vi "CLSUIP_GrowTermBounds.vi"(1 "Center Point":cluster{"x":i32, "y":i32}, 2 "Multiplication Factor":cluster{"x":i32, "y":i32}, 3 "Terminal Bounds":T1) -> (0 "Grown Bounds":T1)   [LabVIEW 2021, in "MemberVICreation.lvlib" / "VIRetooler.lvclass"]
uses:
  <resource>/Framework/Providers/LVClassLibrary/NewAccessors/VIRetooler/VIRetooler.lvclass
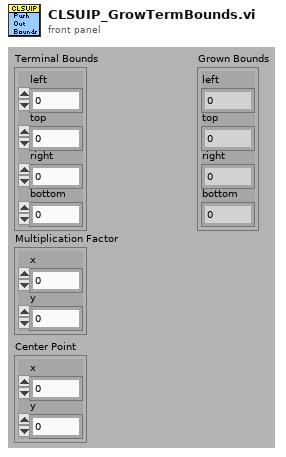
[diagram p1: front panel]
types:
  T1 = cluster{"left":i16, "top":i16, "right":i16, "bottom":i16}
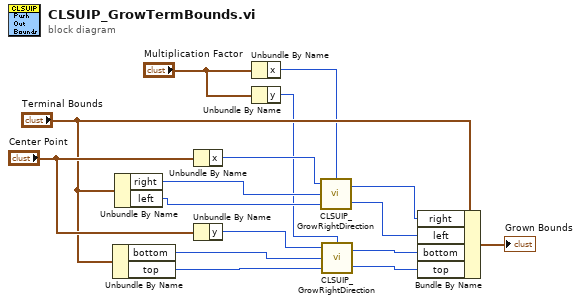
[diagram p0: block diagram]
diagram:
  n1 = Unbundle By Name("Terminal Bounds") -> ("bottom"=w6:i16, "top"=w5:i16)
  n2 = Unbundle By Name("Terminal Bounds") -> ("right"=w10:i16, "left"=w9:i16)
  n3 = Unbundle By Name("Center Point") -> ("x"=w12:i32)
  n4 = Unbundle By Name("Center Point") -> ("y"=w4:i32)
  n5 = Unbundle By Name("Multiplication Factor") -> ("x"=w7:i32)
  n6 = Unbundle By Name("Multiplication Factor") -> ("y"=w3:i32)
  n7 = call <resource>:"CLSUIP_GrowRightDirection.vi"("Multiplication Factor"=w7, "lower"=w9, "higher"=w10, "point"=w12) -> ("new lower"=w8:i16, "new higher"=w11:i16)
  n8 = call <resource>:"CLSUIP_GrowRightDirection.vi"("Multiplication Factor"=w3, "lower"=w5, "higher"=w6, "point"=w4) -> ("new lower"=w1:i16, "new higher"=w2:i16)
  n9 = Bundle By Name(cluster="Terminal Bounds", "right"=w11, "left"=w8, "bottom"=w2, "top"=w1) -> (→"Grown Bounds":T1)
